vi "Delete Float32Array DVR.vi"(8 "error in (no error)":errorcluster, 11 "Float32Array DVR in":refnum<data-value>) -> (0 "error out":errorcluster, 3 "Float32Array out":refnum<class "Float32Array.lvclass">)   [LabVIEW 2015, in "MDSplus.lvlib" / "Float32Array.lvclass"]
uses:
  Float32Array.lvclass
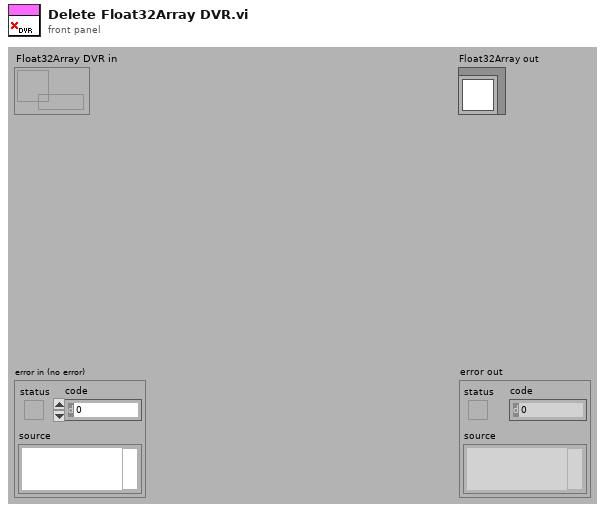
[diagram p1: front panel]
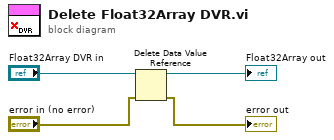
[diagram p0: block diagram]
diagram:
  n1 = Delete Data Value Reference(data value reference="Float32Array DVR in", error in="error in (no error)") -> (data value=→"Float32Array out":refnum<class "Float32Array.lvclass">, error out=→"error out":errorcluster)
